vi "statisticsUI.vi"(11 "StatisticsDisplay in":refnum<class "StatisticsDisplay.lvclass">) -> ()   [LabVIEW 2018, in "StatisticsDisplay.lvclass"]
uses:
  StatisticsDisplay.lvclass
panel:
  out "StatisticsDisplay out":refnum<class "StatisticsDisplay.lvclass">
  out "Humidity":dbl format="%#_2f%"
  out "Pressure":dbl format="%#_2f atm"
  out "Temperature":dbl format="%#_2f°C"
  out "error out":errorcluster
  in  "error in (no error)":errorcluster
  # "Statistics Display"
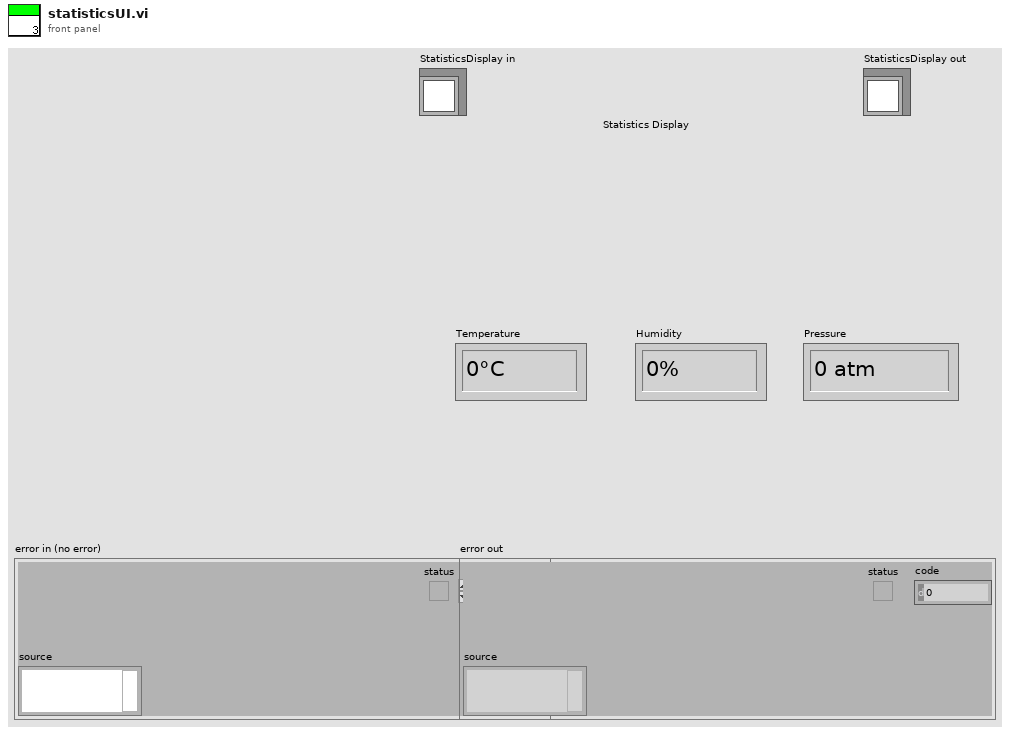
[diagram p1: front panel]
types:
  T1 = enum16{"Always On", "Always Off", "Off While Running"}
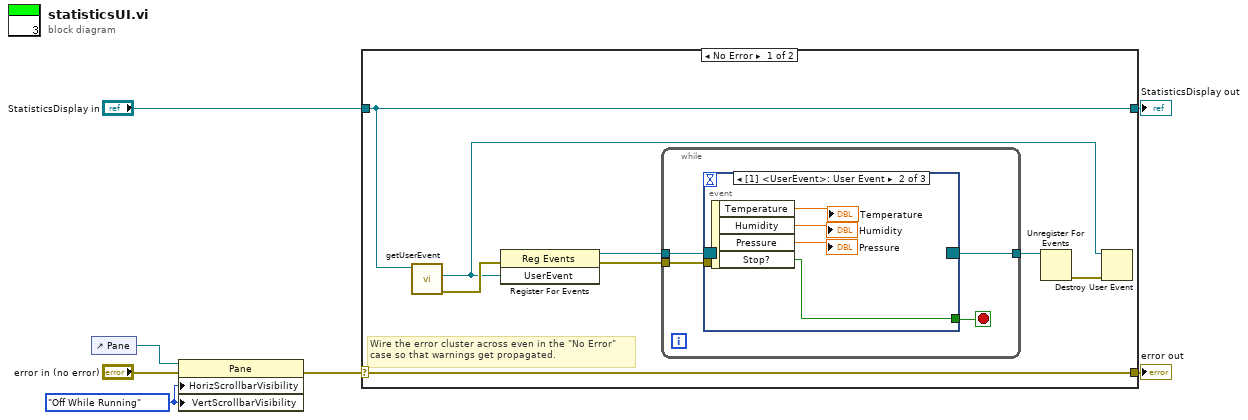
[diagram p0: block diagram]
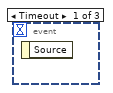
[diagram p2: hidden frame]
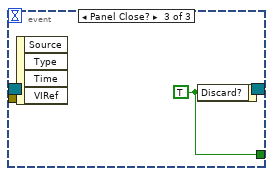
[diagram p3: hidden frame]
diagram:
  w2 = T1."Off While Running" ("Vertical Scrollbar Visibility")
  n1 = control-ref of="Pane"() -> (w1:refnum<vi>)
  n2 = property class="Pane"(reference=w1, error in="error in (no error)", "HorizScrollbarVisibility"=w2, "VertScrollbarVisibility"=w2) -> (error out=w3:errorcluster)  [unwired: 1 out]
  n3 = case shown="No Error" w3 {
    selector: w3 -> [w15 w26]
    tunnel: [w15 w26] -> w6
    tunnel: [w8 w25] -> w4
    tunnel: "StatisticsDisplay in" -> [w8 w25]
    frame No Error {
      # "Wire the error cluster across even in the \"No Error\"\ncase so that warnings get propagated."
      n4 = call-dynamic "getUserEvent.vi"("StatisticsDisplay in"=w8) -> ("error out"=w13:errorcluster, "UserEvent"=w9:refnum<user-event>)  [unwired: 8 in, 1 out]
      n5 = register-events(error in=w13, w9) -> (reference out=w14:refnum<event-registration>, error out=w12:errorcluster)  [unwired: 1 in]
      n6 = while {
        tunnel: w14 -> [w19]
        tunnel: w12 -> [w18]
        tunnel: [w16] -> w11
        stop <- w17 stop-if-true
        n7 = event shown="[1] <UserEvent>: User Event" {
          selector: w19 -> [_ _ _]
          dyn-events: [_ _ _] -> w16
          timeout: _ -> [_ _ _]
          tunnel: w18 -> [_ _ _]
          tunnel: [_ w20 w24] -> w17
          event Timeout {
            n8 = event-data() -> ()  [unwired: 1 in, 1 out]
          }
          event User Event {
            n9 = event-data() -> ("Temperature"=→"Temperature":dbl, "Humidity"=→"Humidity":dbl, "Pressure"=→"Pressure":dbl, "Stop?"=w20:bool)  [unwired: 1 in]
          }
          event Panel Close? {
            w24 = TRUE ("Discard?")
            n10 = event-data() -> ()  [unwired: 1 in, 4 out]
            n11 = event-data("Discard?"=w24) -> ()  [unwired: 1 in, 1 out]
          }
        }
      }
      n12 = Unregister For Events(event registration refnum=w11) -> (error out=w10:errorcluster)  [unwired: 1 in]
      n13 = Destroy User Event(user event=w9, error in=w10) -> ()  [unwired: 1 out]
    }
    frame Error {
    }
  }
  "error out" <- w6
  "StatisticsDisplay out" <- w4
